vi "Gen_TrajLib_Doc.vi"() -> ()   [LabVIEW 2019]
doc: "Generates and HTML file with the Description of every class, library, ctl, and vi in every open project. Creates separate documents for each library and virtual folder , and links to the top level document. In addition, for every VI shows connector pane. Saves the HTML file in folder <project folder>\\<project name> Documentation\\Documentation.html. erases previous content if any. \nDoes not create documentation for Documentation folder in project if exists. Does not create documentation for packed libraries in the project."
uses:
  Doc_Builder_SubVI/FileAndPath.ctl
  <vilib>/Utility/NIReport.llb/NI_report.lvclass
panel:
  in  "Finished":bool
  out "ParamFoundBits":u32
  out "application name":string
  out "Cmd Line Read Error":errorcluster
  out "arguments":string[](array[string])
  in  "Group Name is \nSecond Part of \nFile Name":bool
  in  "Use Second Input\nLibrary":bool=TRUE
  out "Resolved Input Library Path":path
  out "Resolved Input Library 2 Path":path
  out "Current Section":string
  in  "Input Library Path 2":path=path "../../FRC_LV_Trajectory_Library/VI"
  out "File Index":i32
  out "File Count":i32
  in  "stop":bool
  out "Full Input File Name":path
  in  "GO":bool
  in  "Output Documentation Path":path=path "../HTML_Build_Work/Temp"
  in  "Input Library Path":path=path "../../FRC_LV_Trajectory_Library"
  out "Resolved Output Documentation Path":path
  # "DOCUMENT VI"
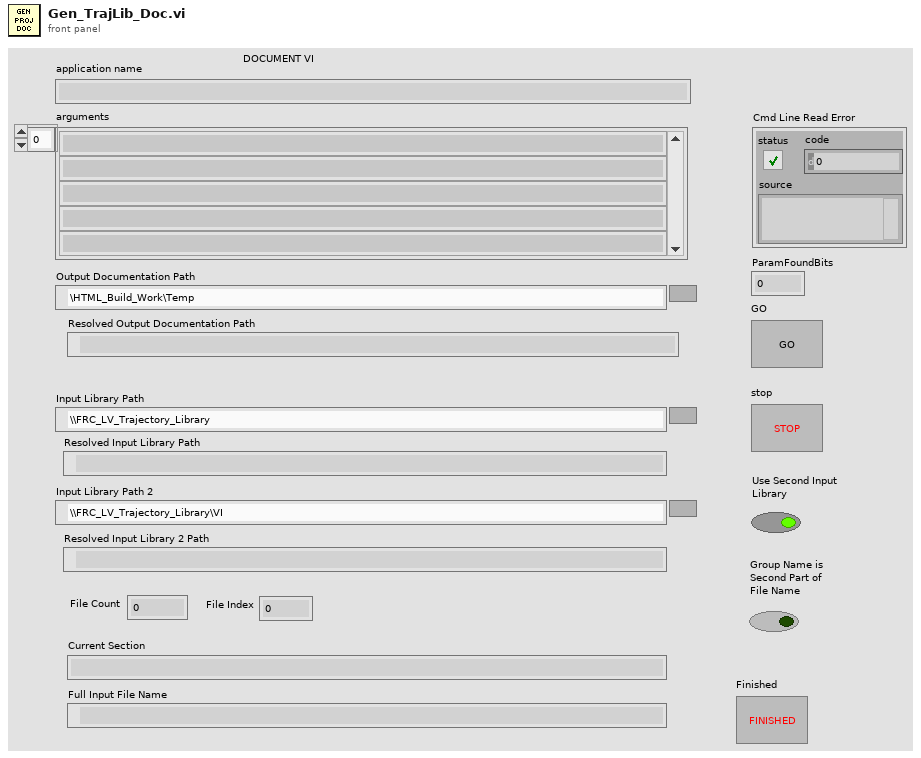
[diagram p1: front panel]
types:
  T1 = typedef "FileAndPath.ctl" = cluster{"FileName":string, "Library Path":path}
  T2 = enum16{"Standard Report", "HTML", "Word", "Excel"}
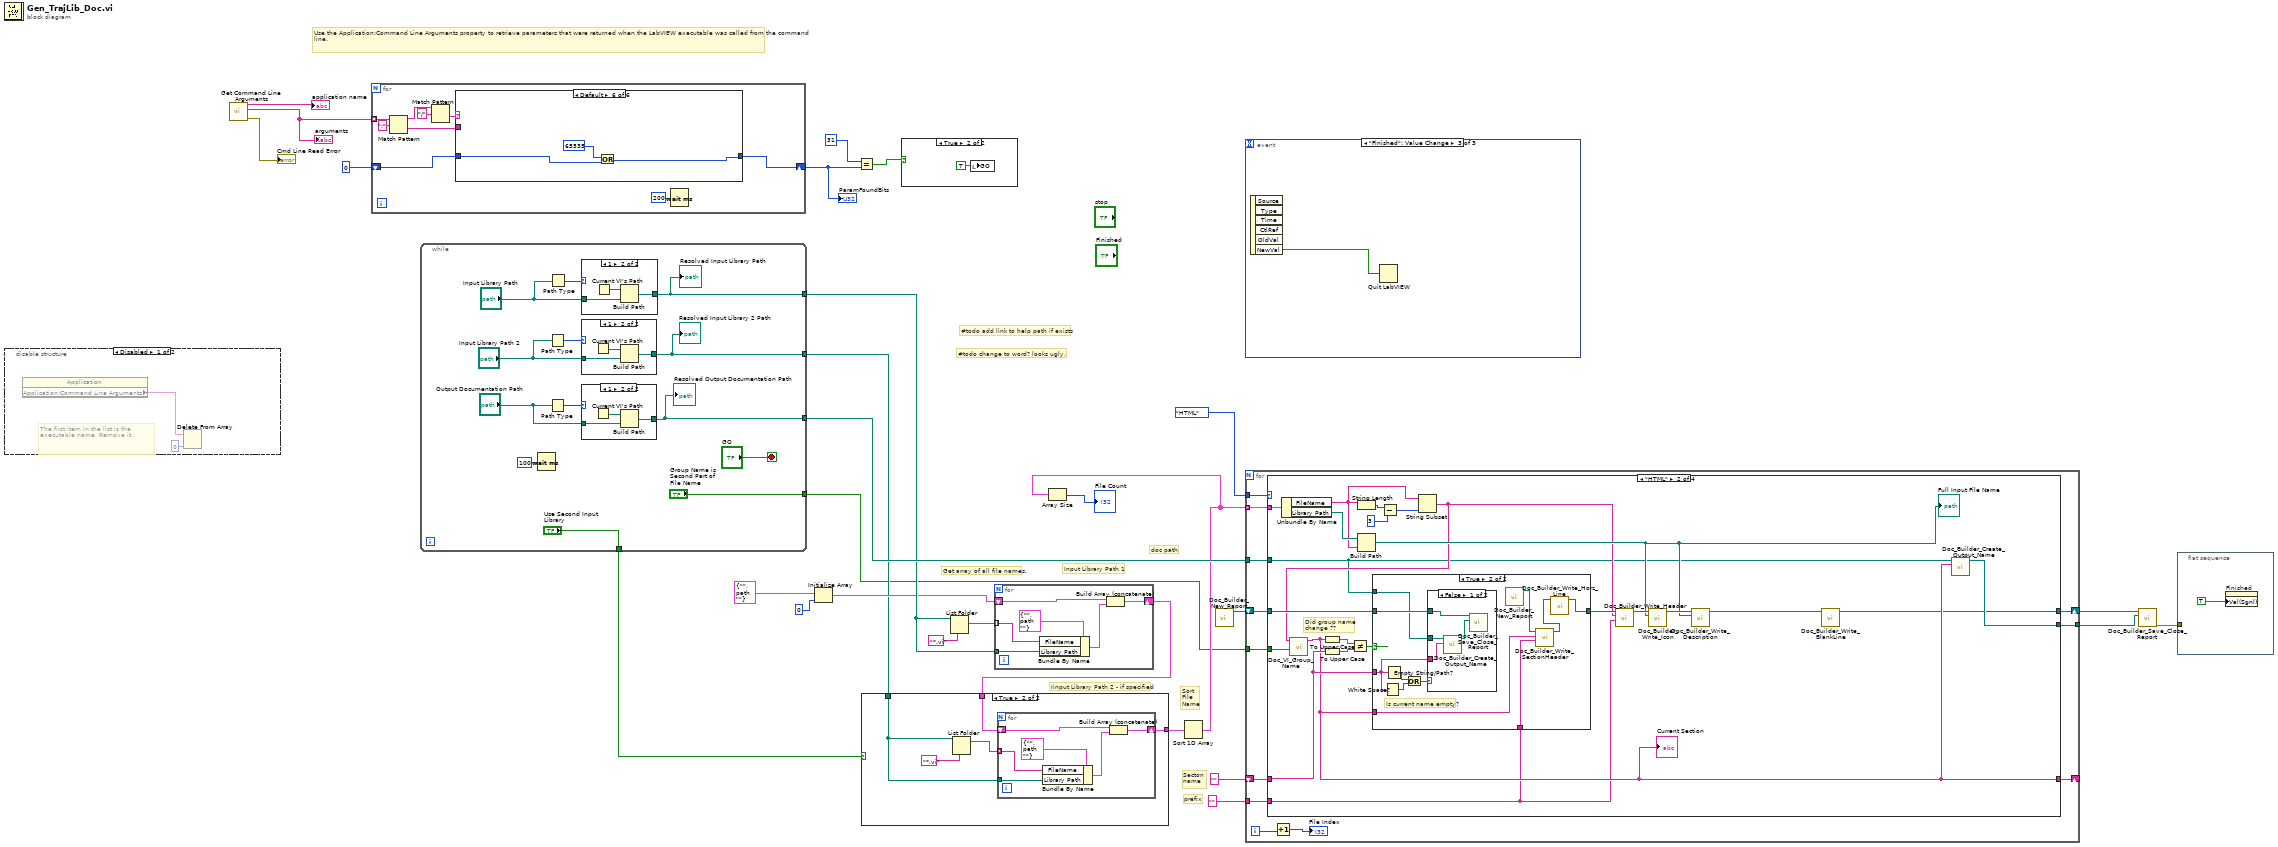
[diagram p0: block diagram]
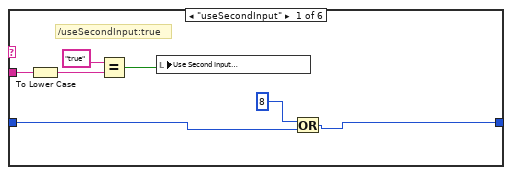
[diagram p4: hidden frame]
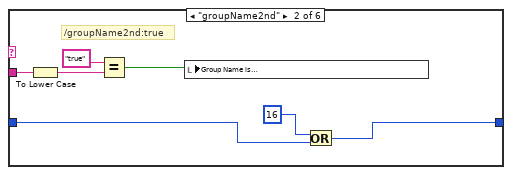
[diagram p5: hidden frame]
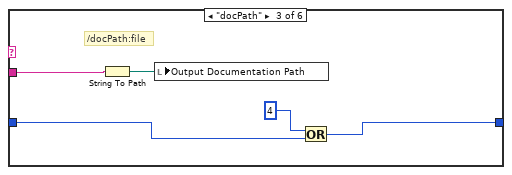
[diagram p6: hidden frame]
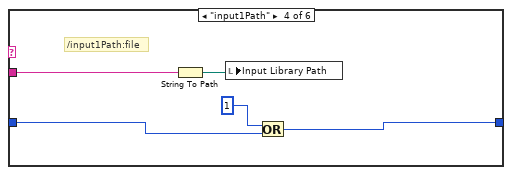
[diagram p7: hidden frame]
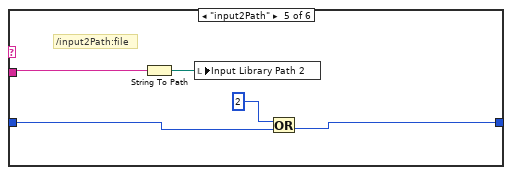
[diagram p8: hidden frame]
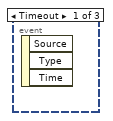
[diagram p10: hidden frame]
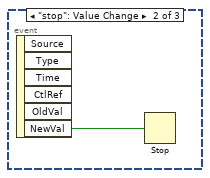
[diagram p11: hidden frame]
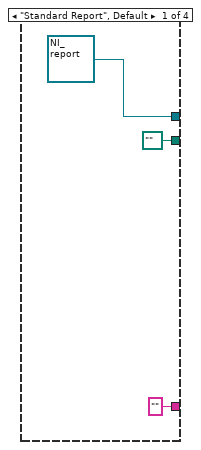
[diagram p15: hidden frame]
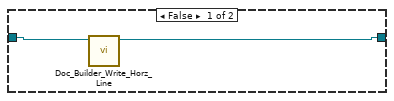
[diagram p16: hidden frame]
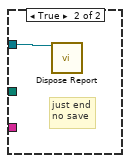
[diagram p17: hidden frame]
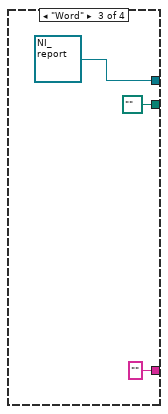
[diagram p18: hidden frame]
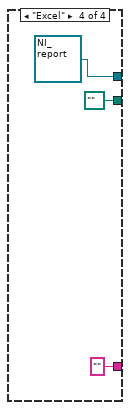
[diagram p19: hidden frame]
diagram:
  # "doc path"
  # "Sort\nFile\nName"
  # "Get array of all file names."
  # "Iinput Library Path 2 - if specified"
  # "Use the Application:Command Line Arguments property to retrieve parameters that were returned when the LabVIEW executable was called from the command line."
  # "Input Library Path 1"
  # "Secton \nname"
  # "prefix"
  # "#todo change to word? looks ugly."
  # "#todo add link to help path if exists"
  n1 = disable-structure shown="Disabled" {
    frame Disabled {
      # "The first item in the list is the executable name. Remove it."
      n2 = property class="Application"() -> ("Application:Command Line Arguments"=w30:string[])  [unwired: 2 in, 2 out]
      n3 = Delete From Array(array=w30, index=0 ("length")) -> ()  [unwired: 1 in, 2 out]
    }
    frame Enabled {
    }
  }
  n4 = call <vilib>:"Get Command Line Arguments.vi"() -> ("error out"=→"Cmd Line Read Error":errorcluster, "arguments"=w4:string[], "application name"=→"application name":string)  [unwired: 9 in]
  "arguments" <- w4
  n5 = for {
    tunnel: w4 -> [w38] mode=indexing
    shift-right: [w32] -> w3
    shift-left: u32 0 -> [w33]
    n6 = Match Pattern(string=w38, regular expression=":") -> (before substring=w36:string, after substring=w37:string)  [unwired: 3 out]
    n7 = Match Pattern(string=w36, regular expression="/") -> (after substring=w34:string)  [unwired: 4 out]
    n8 = case shown="Default" w34 {
      tunnel: w37 -> [w45 w52 w57 w62 w67 _]
      tunnel: [w40 w47 w54 w60 w64 w69] -> w32
      tunnel: w33 -> [w41 w48 w55 w61 w65 w70]
      frame "useSecondInput" {
        # "/useSecondInput:true"
        n9 = To Lower Case(string=w45) -> (all lower case string=w44:string)
        n10 = Equal?(x="true", y=w44) -> (x = y?=w43:bool)
        n11 = local write "Use Second Input\nLibrary"(w43) -> ()
        n12 = Or(x=u32 8, y=w41) -> (x .or. y?=w40:u32)
      }
      frame "groupName2nd" {
        # "/groupName2nd:true"
        n13 = To Lower Case(string=w52) -> (all lower case string=w51:string)
        n14 = Equal?(x="true", y=w51) -> (x = y?=w50:bool)
        n15 = local write "Group Name is \nSecond Part of \nFile Name"(w50) -> ()
        n16 = Or(x=u32 16, y=w48) -> (x .or. y?=w47:u32)
      }
      frame "docPath" {
        # "/docPath:file"
        n17 = String To Path(string=w57) -> (path=w58:path)
        n18 = local write "Output Documentation Path"(w58) -> ()
        n19 = Or(x=u32 4, y=w55) -> (x .or. y?=w54:u32)
      }
      frame "input1Path" {
        # "/input1Path:file"
        n20 = String To Path(string=w62) -> (path=w63:path)
        n21 = local write "Input Library Path"(w63) -> ()
        n22 = Or(x=u32 1, y=w61) -> (x .or. y?=w60:u32)
      }
      frame "input2Path" {
        # "/input2Path:file"
        n23 = String To Path(string=w67) -> (path=w68:path)
        n24 = local write "Input Library Path 2"(w68) -> ()
        n25 = Or(x=u32 2, y=w65) -> (x .or. y?=w64:u32)
      }
      frame Default {
        n26 = Or(x=u32 65535, y=w70) -> (x .or. y?=w69:u32)
      }
    }
    n27 = Wait (ms)(milliseconds to wait=u32 200) -> ()  [unwired: 1 out]
  }
  "ParamFoundBits" <- w3
  n28 = while {
    tunnel: [w82] -> w26
    tunnel: [w74] -> w22
    tunnel: [w75] -> w17
    tunnel: ["Group Name is \nSecond Part of \nFile Name"] -> w9
    tunnel: ["Use Second Input\nLibrary"] -> w8
    stop <- "GO" stop-if-true
    n29 = Wait (ms)(milliseconds to wait=u32 100) -> ()  [unwired: 1 out]
    n30 = Path Type(1:"Input Library Path 2") -> (0:w79:i16)
    n31 = Path Type(1:"Output Documentation Path") -> (0:w80:i16)
    n32 = Path Type(1:"Input Library Path") -> (0:w77:i16)
    n33 = case shown="1" w79 {
      tunnel: [w89 w91] -> w75
      tunnel: "Input Library Path 2" -> [w89 w90]
      frame 0, Default {
      }
      frame 1 {
        n34 = Current VI's Path() -> (path=w92:path)
        n35 = Build Path(base path=w92, name or relative path=w90) -> (appended path=w91:path)
      }
    }
    "Resolved Input Library 2 Path" <- w75
    n36 = case shown="1" w80 {
      tunnel: [w93 w95] -> w82
      tunnel: "Output Documentation Path" -> [w93 w94]
      frame 0, Default {
      }
      frame 1 {
        n37 = Current VI's Path() -> (path=w96:path)
        n38 = Build Path(base path=w96, name or relative path=w94) -> (appended path=w95:path)
      }
    }
    "Resolved Output Documentation Path" <- w82
    n39 = case shown="1" w77 {
      tunnel: [w85 w87] -> w74
      tunnel: "Input Library Path" -> [w85 w86]
      frame 0, Default {
      }
      frame 1 {
        n40 = Current VI's Path() -> (path=w88:path)
        n41 = Build Path(base path=w88, name or relative path=w86) -> (appended path=w87:path)
      }
    }
    "Resolved Input Library Path" <- w74
  }
  n42 = Initialize Array(T1 {"FileName"="", "Library Path"=path ""} ("FileAndPath"), 0 ("dimension size")) -> (w20:T1[])
  n43 = Equal?(x=u32 31, y=w3) -> (x = y?=w1:bool)
  n44 = case shown="True" w1 {
    frame False {
    }
    frame True {
      n45 = local write "GO"(TRUE ("GO")) -> ()
    }
  }
  n46 = List Folder(path=w22, pattern="*.vi") -> (filenames=w23:string[])  [unwired: 2 in, 3 out]
  n47 = for {
    tunnel: w23 -> [w103] mode=indexing
    tunnel: w22 -> [w102]
    shift-right: [w101] -> w18
    shift-left: w20 -> [w100]
    n48 = Bundle By Name(cluster=T1 {"FileName"="", "Library Path"=path ""} ("FileAndPath"), "FileName"=w103, "Library Path"=w102) -> (w98:T1)
    n49 = Build Array (concatenate)(w100, w98) -> (w101:T1[])
  }
  n50 = case shown="True" w8 {
    tunnel: w18 -> [w104 w108]
    tunnel: w17 -> [_ w106]
    tunnel: [w104 w105] -> w16
    frame False {
    }
    frame True {
      n51 = List Folder(path=w106, pattern="*.vi") -> (filenames=w107:string[])  [unwired: 2 in, 3 out]
      n52 = for {
        tunnel: w107 -> [w115] mode=indexing
        tunnel: w106 -> [w114]
        shift-right: [w113] -> w105
        shift-left: w108 -> [w112]
        n53 = Bundle By Name(cluster=T1 {"FileName"="", "Library Path"=path ""} ("FileAndPath"), "FileName"=w115, "Library Path"=w114) -> (w110:T1)
        n54 = Build Array (concatenate)(w112, w110) -> (w113:T1[])
      }
    }
  }
  n55 = Sort 1D Array(array=w16) -> (sorted array=w15:T1[])
  n56 = Array Size(array=w15) -> (size(s)=→"File Count":i32)
  n57 = call "Doc_Builder_New_Report.vi"() -> ("NI_report out"=w14:refnum<class "NI_report.lvclass">)  [unwired: 11 in]
  n58 = for {
    tunnel: w15 -> [w126] mode=indexing
    tunnel: T2."HTML" ("report type") -> [w127]
    tunnel: w26 -> [w125]
    tunnel: "" ("string") -> [w122]
    shift-right: [w118] -> w12
    shift-left: w14 -> [w121]
    shift-right: [w117] -> _
    shift-left: "" ("string") -> [w120]
    tunnel: [w119] -> w11
    tunnel: w9 -> [w116]
    i -> [w124]
    n59 = case shown="\"HTML\"" w127 {
      tunnel: w126 -> [_ w148 _ _]
      tunnel: w125 -> [_ w136 _ _]
      tunnel: w122 -> [_ w134 _ _]
      tunnel: w121 -> [_ w141 _ _]
      tunnel: w120 -> [_ w137 _ _]
      tunnel: [path "" ("Full Report Name") w139 path "" ("Full Report Name") path "" ("Full Report Name")] -> w119
      tunnel: [refnum<class "NI_report.lvclass"> refnum ("report out") w132 refnum<class "NI_report.lvclass"> refnum ("report out") refnum<class "NI_report.lvclass"> refnum ("report out")] -> w118
      tunnel: ["" ("FileName") w135 "" ("FileName") "" ("FileName")] -> w117
      tunnel: w116 -> [_ w131 _ _]
      frame "Standard Report", Default {
      }
      frame "HTML" {
        # "Did group name\nchange ??"
        n60 = Unbundle By Name(w148) -> ("FileName"=w146:string, "Library Path"=w147:path)
        n61 = To Upper Case(1:w137) -> (0:w143:string)
        n62 = Build Path(base path=w147, name or relative path=w146) -> (appended path=w145:path)
        "Full Input File Name" <- w145
        n63 = String Length(string=w146) -> (length=w153:i32)
        n64 = Subtract(x=w153, y=3) -> (x-y=w151:i32)
        n65 = String Subset(string=w146, length (rest)=w151) -> (substring=w138:string)  [unwired: 1 in]
        n66 = call "Doc_VI_Group_Name.vi"("Group Name is second\npart of file name"=w131, "FileName"=w138) -> ("Section Name"=w135:string)  [unwired: 9 in]
        "Current Section" <- w135
        n67 = To Upper Case(1:w135) -> (0:w144:string)
        n68 = Not Equal?(x=w144, y=w143) -> (x != y?=w142:bool)
        n69 = case shown="True" w142 {
          tunnel: w141 -> [w155 w163]
          tunnel: [w154 w160] -> w140
          tunnel: w137 -> [_ w161]
          tunnel: w136 -> [_ w162]
          tunnel: w135 -> [_ w157]
          tunnel: w134 -> [_ w156]
          frame False {
            n70 = call "Doc_Builder_Write_Horz_Line.vi"("NI_report in"=w155) -> ("NI_report out"=w154:refnum<class "NI_report.lvclass">)  [unwired: 10 in]
          }
          frame True {
            # "Is current name empty?"
            n71 = White Space?(1:w161) -> (0:w165:bool)
            n72 = Empty String/Path?(string/path=w161) -> (empty?=w164:bool)
            n73 = Or(x=w164, y=w165) -> (x .or. y?=w166:bool)
            n74 = case shown="False" w166 {
              tunnel: w163 -> [w170 w171]
              tunnel: w162 -> [w169 _]
              tunnel: w161 -> [w168 _]
              frame False {
                n75 = call "Doc_Builder_Create_Output_Name.vi"("Section Name"=w168, "Path"=w169) -> ("Full Report Name"=w167:path)  [unwired: 9 in]
                n76 = call "Doc_Builder_Save_Close_Report.vi"("appended path"=w167, "NI_report in"=w170) -> ()  [unwired: 9 in, 1 out]
              }
              frame True {
                # "just end\nno save"
                n77 = call-dynamic "Dispose Report.vi"("report in"=w171) -> ()  [unwired: 14 in, 1 out]
              }
            }
            n78 = call "Doc_Builder_New_Report.vi"() -> ("NI_report out"=w159:refnum<class "NI_report.lvclass">)  [unwired: 11 in]
            n79 = call "Doc_Builder_Write_SectionHeader.vi"("Prefix String"=w156, "Section Name"=w157, "NI_report in"=w159) -> ("NI_report out"=w158:refnum<class "NI_report.lvclass">)  [unwired: 8 in]
            n80 = call "Doc_Builder_Write_Horz_Line.vi"("NI_report in"=w158) -> ("NI_report out"=w160:refnum<class "NI_report.lvclass">)  [unwired: 10 in]
          }
        }
        n81 = call "Doc_Builder_Write_Header.vi"("Prefix String"=w134, "Item Name"=w138, "NI_report in"=w140) -> ("NI_report out"=w150:refnum<class "NI_report.lvclass">)  [unwired: 8 in]
        n82 = call "Doc_Builder_Write_Icon.vi"("Input Item file path"=w145, "NI_report in"=w150) -> ("NI_report out"=w149:refnum<class "NI_report.lvclass">)  [unwired: 9 in]
        n83 = call "Doc_Builder_Write_Description.vi"("input item file path"=w145, "NI_report in"=w149) -> ("NI_report out"=w133:refnum<class "NI_report.lvclass">)  [unwired: 9 in]
        n84 = call "Doc_Builder_Write_BlankLine.vi"("NI_report in"=w133) -> ("NI_report out"=w132:refnum<class "NI_report.lvclass">)  [unwired: 10 in]
        n85 = call "Doc_Builder_Create_Output_Name.vi"("Section Name"=w135, "Path"=w136) -> ("Full Report Name"=w139:path)  [unwired: 9 in]
      }
      frame "Word" {
      }
      frame "Excel" {
      }
    }
    n86 = Increment(x=w124) -> (x+1=→"File Index":i32)
  }
  n87 = event shown="[2] \"Finished\": Value Change" {
    selector: _ -> [_ _ _]
    dyn-events: _ -> [_ _ _]
    timeout: _ -> [_ _ _]
    event Timeout {
      n88 = event-data() -> ()  [unwired: 1 in, 3 out]
    }
    event "stop": Value Change {
      n89 = event-data() -> ("NewVal"=w178:bool)  [unwired: 1 in, 5 out]
      n90 = Stop(stop? (T)=w178) -> ()
    }
    event "Finished": Value Change {
      n91 = event-data() -> ("NewVal"=w179:bool)  [unwired: 1 in, 5 out]
      n92 = Quit LabVIEW(quit? (T)=w179) -> ()
    }
  }
  n93 = call "Doc_Builder_Save_Close_Report.vi"("appended path"=w11, "NI_report in"=w12) -> ("error out"=w10:errorcluster)  [unwired: 9 in]
  n94 = flat-sequence {
    tunnel: w10 -> [_]
    frame #0 {
      n95 = property on="Finished" class="Bool (strict)"("Val(Sgnl)"=TRUE ("Finished")) -> ()  [unwired: 2 in, 2 out]
    }
  }
